vi "T controller.vi"() -> ()   [LabVIEW 2017]
uses:
  <instrlib>/Lake Shore 335/Lake Shore 335.lvlib
panel:
  in  "Tab Control":enum32{"Page 1", "Page 2"}(tab)
  in  "T 2":dbl[](array[numeric])
  out "T":cluster{"Sensor Data":dbl, "Sensor Data":dbl}(graph)
  out "Heater (%)":dbl format="%.1f"
  in  "Set":dbl format="%.4f"
  out "n":dbl
  out "m":dbl
  in  "Ramp Rate (0.0)":dbl=10.0 format="%.1f"
  in  "Ramping":bool=TRUE
  in  "stop":bool
  in  "VISA resource name":refnum<visa-resource-name>="GPIB0::12::INSTR"
  out "VISA resource name out":refnum<visa-resource-name>
  in  "set":bool
  in  "error in (no error)":errorcluster
  out "error out":errorcluster
  in  "Output's Control Loop (1:1)":u16(ring)=1 items=["1"=1, "2"=2]
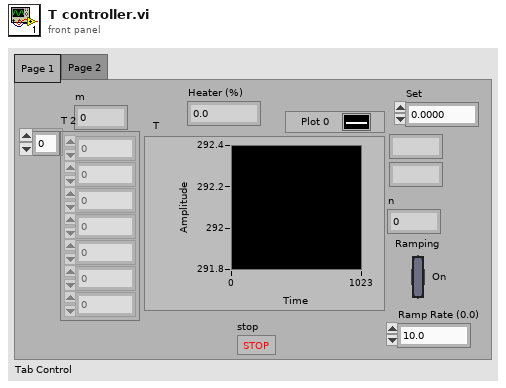
[diagram p1: front panel]
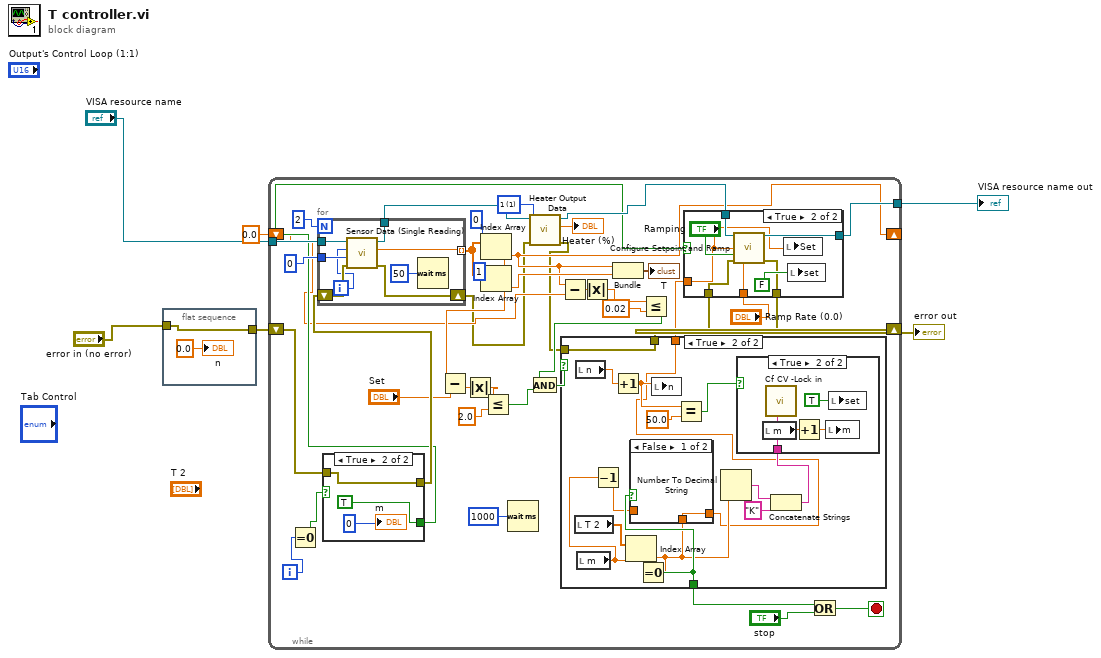
[diagram p0: block diagram]
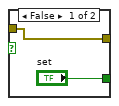
[diagram p2: hidden frame]
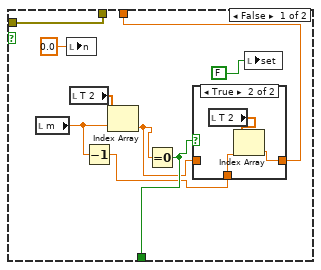
[diagram p3: hidden frame]
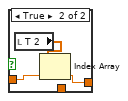
[diagram p5: hidden frame]
diagram:
  n1 = flat-sequence {
    tunnel: "error in (no error)" -> [w7]
    tunnel: [w7] -> w2
    frame #0 {
      "n" <- 0.0 ("n")
    }
  }
  n2 = while {
    tunnel: "VISA resource name" -> [w38]
    shift-right: [w36] -> w5
    shift-left: w2 -> [w29]
    tunnel: [w37] -> w4
    shift-right: [w20] -> _
    shift-left: 0.0 ("Sensor Data") -> [w19]
    i -> [w27]
    stop <- w15 stop-if-true
    w40 = u16 1 items=["1"=1, "2"=2] ("Heater Output (1:1)")
    n3 = Equal To 0?(x=w27) -> (x = 0?=w26:bool)
    n4 = case shown="True" w26 {
      tunnel: w29 -> [w50 w53]
      tunnel: [w50 w53] -> w28
      tunnel: ["set" TRUE ("set")] -> w21
      frame False {
      }
      frame True {
        "m" <- 0
      }
    }
    n5 = for {
      N: 2 -> [_]
      tunnel: w38 -> [w105]
      tunnel: 0 -> [w104]
      shift-right: [w103] -> w14
      shift-left: w28 -> [w106]
      tunnel: [w100] -> w46 mode=indexing
      tunnel: [w101] -> w41
      i -> [w102]
      n6 = call "Sensor Data (Single Reading).vi"("error in (no error)"=w106, "Data Source (0:Kelvin)"=w104, "Input (0:A)"=w102, "VISA resource name"=w105) -> ("error out"=w103:errorcluster, "Sensor Data"=w100:dbl, "VISA resource name out"=w101:refnum<visa-resource-name>)  [unwired: 5 in]
      n7 = Wait (ms)(milliseconds to wait=u32 50) -> ()  [unwired: 1 out]
    }
    n8 = Index Array(array=w46, index=0) -> (element=w20:dbl)
    n9 = Subtract(x=w20, y="Set") -> (x-y=w10:dbl)
    n10 = Absolute Value(x=w10) -> (abs(x)=w9:dbl)
    n11 = Index Array(array=w46, index=1) -> (element=w33:dbl)
    n12 = Less Or Equal?(x=w9, y=2.0) -> (x <= y?=w11:bool)
    n13 = Wait (ms)(milliseconds to wait=u32 1000) -> ()  [unwired: 1 out]
    n14 = call "Heater Output Data.vi"("error in (no error)"=w14, "Heater Output (1:1)"=w40, "VISA resource name"=w41) -> ("error out"=w13:errorcluster, "Output Value"=→"Heater (%)":dbl, "VISA resource name out"=w22:refnum<visa-resource-name>)  [unwired: 6 in]
    n15 = Subtract(x=w20, y=w19) -> (x-y=w35:dbl)
    n16 = Absolute Value(x=w35) -> (abs(x)=w18:dbl)
    n17 = Bundle("Sensor Data"=w20, "Sensor Data"=w33) -> (→"T":cluster{"Sensor Data":dbl, "Sensor Data":dbl})  [unwired: 1 in]
    n18 = Less Or Equal?(x=w18, y=0.02) -> (x <= y?=w25:bool)
    n19 = And(x=w25, y=w11) -> (x .and. y?=w24:bool)
    n20 = case shown="True" w24 {
      tunnel: w13 -> [w61 w72]
      tunnel: [w61 w72] -> w32
      tunnel: [w56 w67] -> w30
      tunnel: [w58 w71] -> w17
      frame False {
        n21 = local read "m"() -> (w55:dbl)
        n22 = local write "n"(0.0 ("n")) -> ()
        n23 = local read "T 2"() -> (w60:dbl[])
        n24 = Decrement(x=w55) -> (x-1=w54:dbl)
        n25 = Index Array(array=w60, index=w55) -> (element=w57:dbl)
        n26 = Equal To 0?(x=w57) -> (x = 0?=w58:bool)
        n27 = case shown="True" w58 {
          tunnel: w57 -> [w63 _]
          tunnel: [w63 w65] -> w56
          tunnel: w54 -> [_ w64]
          frame False {
          }
          frame True {
            n28 = local read "T 2"() -> (w66:dbl[])
            n29 = Index Array(array=w66, index=w64) -> (element=w65:dbl)
          }
        }
        n30 = local write "set"(FALSE) -> ()
      }
      frame True {
        n31 = local read "T 2"() -> (w76:dbl[])
        n32 = local read "n"() -> (w80:dbl)
        n33 = local read "m"() -> (w70:dbl)
        n34 = Decrement(x=w70) -> (x-1=w69:dbl)
        n35 = Increment(x=w80) -> (x+1=w79:dbl)
        n36 = Index Array(array=w76, index=w70) -> (element=w68:dbl)
        n37 = Equal To 0?(x=w68) -> (x = 0?=w71:bool)
        n38 = case shown="False" w71 {
          tunnel: w69 -> [_ w82]
          tunnel: [w81 w83] -> w67
          tunnel: w68 -> [w81 _]
          frame False {
          }
          frame True {
            n39 = local read "T 2"() -> (w84:dbl[])
            n40 = Index Array(array=w84, index=w82) -> (element=w83:dbl)
          }
        }
        n41 = local write "n"(w79) -> ()
        n42 = Equal?(x=w79, y=50.0) -> (x = y?=w77:bool)
        n43 = Number To Decimal String(number=w68) -> (decimal integer string=w75:string)  [unwired: 1 in]
        n44 = Concatenate Strings(w75, "K" ("string")) -> (w73:string)
        n45 = case shown="True" w77 {
          tunnel: w73 -> [_ w88]
          frame False {
          }
          frame True {
            n46 = local read "m"() -> (w87:dbl)
            n47 = call "Cf CV -Lock in.vi"("name"=w88) -> ()  [unwired: 10 in, 1 out]
            n48 = Increment(x=w87) -> (x+1=w86:dbl)
            n49 = local write "m"(w86) -> ()
            n50 = local write "set"(TRUE ("set")) -> ()
          }
        }
      }
    }
    n51 = case shown="True" w21 {
      tunnel: w30 -> [_ w91]
      tunnel: w22 -> [w90 w97]
      tunnel: [w90 w96] -> w37
      tunnel: w32 -> [w89 w94]
      tunnel: [w89 w93] -> w36
      tunnel: "Ramp Rate (0.0)" -> [_ w92]
      frame False {
      }
      frame True {
        n52 = call "Configure Setpoint and Ramp.vi"("VISA resource name"=w97, "Setpoint (0.0000)"=w91, "Enable Setpoint Ramping (F: Off)"="Ramping", "error in (no error)"=w94, "Ramp Rate (0.0)"=w92) -> ("VISA resource name out"=w96:refnum<visa-resource-name>, "error out"=w93:errorcluster)  [unwired: 9 in]
        n53 = local write "Set"(w91) -> ()
        n54 = local write "set"(FALSE) -> ()
      }
    }
    n55 = Or(x=w17, y="stop") -> (x .or. y?=w15:bool)
  }
  "VISA resource name out" <- w4
  "error out" <- w5
